vi "comparison ok.vi"() -> ()   [LabVIEW 2017]
panel:
  out "Boolean":bool
  in  "Numeric 2":i32
  in  "Numeric":dbl
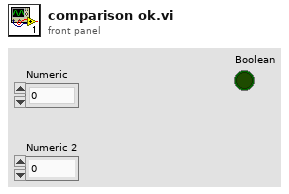
[diagram p1: front panel]
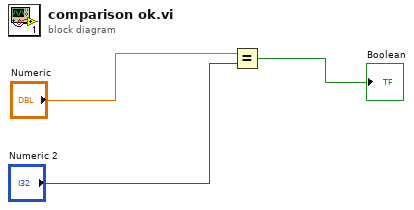
[diagram p0: block diagram]
diagram:
  n1 = Equal?(x="Numeric", y="Numeric 2") -> (x = y?=→"Boolean":bool)
